vi "analog_cache.vi"(1 "Cluster":T1) -> (0 "$_val":fxp<+/-,24,5>)   [LabVIEW 2018]
uses:
  validated_analog.ctl
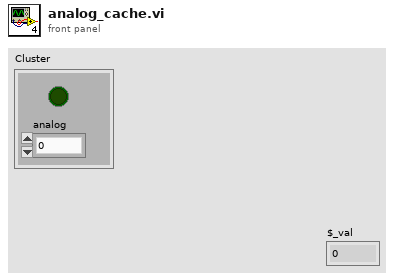
[diagram p1: front panel]
types:
  T1 = typedef "validated_analog.ctl" = cluster{"valid":bool, "analog":fxp<+/-,24,5>}
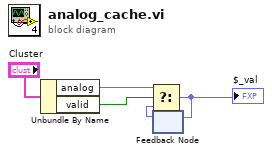
[diagram p0: block diagram]
diagram:
  n1 = Unbundle By Name("Cluster") -> ("analog"=w2:fxp<+/-,24,5>, "valid"=w1:bool)
  n2 = feedback #1() -> (w4:fxp<+/-,24,5>)  [unwired: 1 in]
  n3 = Select(t=w2, s=w1, f=w4) -> (s? t:f=w5:fxp<+/-,24,5>)
  "$_val" <- w5
  n4 = feedback-in #1(w5) -> ()
